vi "Create Report (strict-JUnit).vi.vi"(6 "Verbose":bool, 8 "error in (no error)":errorcluster, 10 "Report Path":path, 11 "strict-JUnit in":refnum<class "strict-JUnit.lvclass">) -> (0 "error out":errorcluster, 3 "strict-JUnit out":refnum<class "strict-JUnit.lvclass">)   [LabVIEW 2013, in "strict-JUnit.lvclass"]
uses:
  strict-JUnit.lvclass
  <vilib>/addons/_JKI Toolkits/Caraya/classes/Test Report/Test Report.lvclass/Test Report.ctl
  <vilib>/addons/_JKI Toolkits/Caraya/classes/Test Report/Test Report.lvclass
  <vilib>/addons/_JKI Toolkits/Caraya/classes/Test Report.JUnit/Test Report.JUnit.lvclass
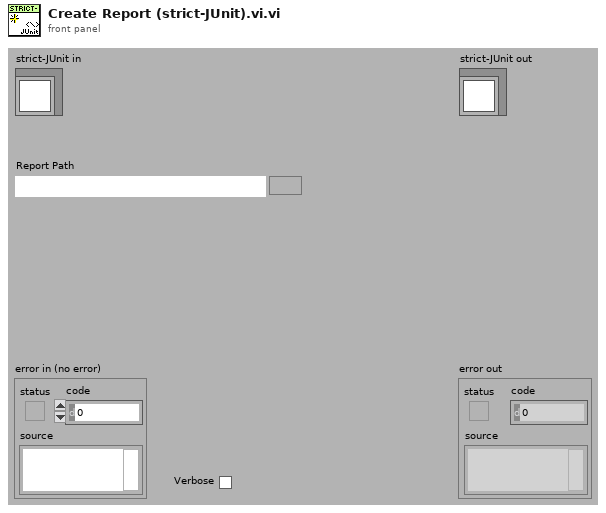
[diagram p1: front panel]
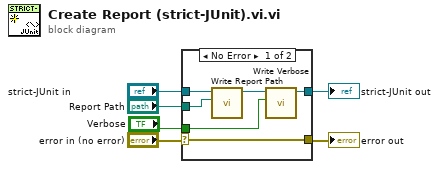
[diagram p0: block diagram]
diagram:
  n1 = case shown="No Error" "error in (no error)" {
    selector: "error in (no error)" -> [w12 w13]
    tunnel: "strict-JUnit in" -> [w9 w14]
    tunnel: [w11 w14] -> w5
    tunnel: "Report Path" -> [w7 _]
    tunnel: [w12 w13] -> w2
    tunnel: "Verbose" -> [w10 _]
    frame No Error {
      n2 = call <vilib>:"Write Report Path.vi"("Report Path"=w7, "Test Report.Default in"=w9) -> ("Test Report.Default out"=w8:refnum<class "strict-JUnit.lvclass">)  [unwired: 9 in]
      n3 = call <vilib>:"Write Verbose.vi"("Verbose"=w10, "Test Report in"=w8) -> ("Test Report out"=w11:refnum<class "strict-JUnit.lvclass">)  [unwired: 8 in, 1 out]
    }
    frame Error {
    }
  }
  "error out" <- w2
  "strict-JUnit out" <- w5
